vi "init.vi"(5 "Scan control":refnum<vi>, 6 "Setup control":refnum<vi>, 7 "Session control":refnum<vi>, 8 "error in (no error)":errorcluster, 10 "Session - Pipeline":path=path "Z:/users/Manolis/Labview/Cajal/Cajal-manolis.dsn", 11 "Experiment in":refnum<class "Experiment.lvclass">) -> (0 "error out":errorcluster, 3 "Experiment out":refnum<class "Experiment.lvclass">)   [LabVIEW 2016, in "Experiment.lvclass"]
uses:
  Experiment.lvclass
  Experiment.lvclass/Experiment.ctl
  Database/Database.lvclass
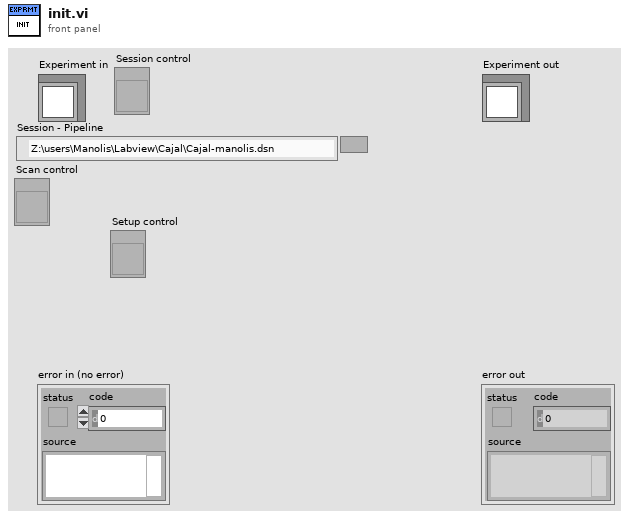
[diagram p1: front panel]
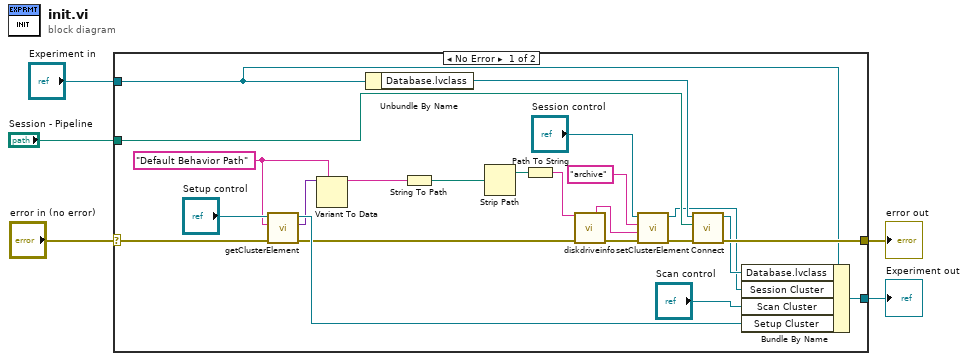
[diagram p0: block diagram]
diagram:
  n1 = case shown="No Error" "error in (no error)" {
    selector: "error in (no error)" -> [w17 w30]
    tunnel: [w27 w30] -> w4
    tunnel: [w23 w29] -> w2
    tunnel: "Experiment in" -> [w25 w29]
    tunnel: "Session - Pipeline" -> [w26 _]
    frame No Error {
      w11 = "Default Behavior Path" ("Label.Text")
      n2 = call "getClusterElement.vi"("error in (no error)"=w17, "Label.Text"=w11, "reference"="Setup control") -> ("error out"=w15:errorcluster, "Value"=w12:variant, "reference 2"=w19:refnum<vi>)  [unwired: 6 in]
      n3 = Variant To Data(type=w11, Variant=w12) -> (data=w9:string)  [unwired: 1 in, 1 out]
      n4 = Unbundle By Name(w25) -> ("Database.lvclass"=w28:refnum<class "Database.lvclass">)
      n5 = String To Path(string=w9) -> (path=w8:path)
      n6 = Strip Path(path=w8) -> (stripped path=w7:path)  [unwired: 1 out]
      n7 = Path To String(path=w7) -> (string=w6:string)
      n8 = call "diskdriveinfo.vi"("Drive Letter"=w6, "error in (no error)"=w15) -> ("drive name"=w10:string, "error out"=w14:errorcluster)  [unwired: 4 in, 8 out]
      n9 = call "setClusterElement.vi"("error in (no error)"=w14, "Value"=w10, "Label.Text"="archive", "reference"="Session control") -> ("error out"=w16:errorcluster, "reference 2"=w18:refnum<vi>)  [unwired: 6 in]
      n10 = call-dynamic "Connect.vi"("error in (no error)"=w16, "Session - Pipeline"=w26, "Database in"=w28) -> ("error out"=w27:errorcluster, "Database out"=w24:refnum<class "Database.lvclass">)  [unwired: 7 in]
      n11 = Bundle By Name(cluster=w25, "Database.lvclass"=w24, "Session Cluster"=w18, "Scan Cluster"="Scan control", "Setup Cluster"=w19) -> (w23:refnum<class "Experiment.lvclass">)
    }
    frame Error {
    }
  }
  "error out" <- w4
  "Experiment out" <- w2
